vi "Test Configure.vi"(0 "Template Rx Test in":refnum<class "niDTS WLAN Rx Test.lvclass">, 11 "error in (no error)":errorcluster) -> (4 "Template Rx Test out":refnum<class "niDTS WLAN Rx Test.lvclass">, 15 "error out":errorcluster)   [LabVIEW 2015, in "niDTS WLAN.lvlib" / "niDTS WLAN Rx Test.lvclass"]
uses:
  niDTS WLAN Rx Test.lvclass
  niDTS WLAN Rx Test.lvclass/niDTS WLAN Rx Test.ctl
  RiviInstDriver/InstDriver/Objects/InstDriver.lvclass/InstDriver.ctl
  RiviInstDriver/InstDriver/Objects/Read VISA resource.vi
  TestStand/Station/Objects/SystemTechnologyCatalog/niDTS SystemTechnologyCatalog.lvclass
  TestStand/Station/Objects/SystemDut/niDTS SystemDut.lvclass
  Framework/Dut/Objects/BASE_class/niDTS Dut.lvclass
  Dut/Objects/BASE_class/niDTS WLAN Dut.lvclass
  Instrument/INSTR RX/niDTS WLAN INSTR RX.lvclass
  niDTS WLAN.lvlib
  Framework/niDTS Framework.lvlib
  RiviInstDriver/niRfsgWlan/Objects/niRfsgWlan.lvclass
  TestStand/niDTS TestStand.lvlib
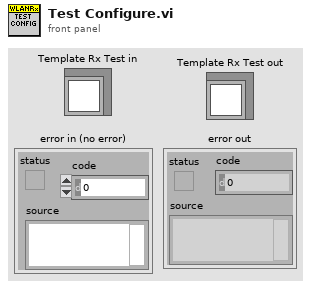
[diagram p1: front panel]
types:
  T1 = typedef "niDTS Framework.lvlib/niDTS Dut INC Handle.ctl" = refnum<data-value>
  T2 = typedef "niDTS WLAN.lvlib/niDTS WLAN Rx Test INC Parameters.ctl" = cluster{"Standard":T3, "DSSS Data Rate (Mbps)":T4, "OFDM Data Rate (Mbps)":T5, "MCS Index":i32, "N Spatial Streams":i32, "Chains":bool[], "Bandwidth (Hz)":T6, "Channel":i32, "Power (dBm)":dbl, "Guard Interval":T7, "FEC Coding":T8, "16 symbols":bool, "Payload Length (bytes)":i32, "Idle Interval (s)":dbl, "External Attenuation (dB)":dbl[], "RX Measurement Parameters":T9}
  T3 = typedef "niDTS WLAN.lvlib/niDTS WLAN INC Standard.ctl" = enum16{"802.11 b DSSS", "802.11 a/g OFDM", "802.11 n HT", "802.11 ac VHT"}
  T4 = typedef "niDTS WLAN.lvlib/niDTS WLAN INC DSSS Data Rate.ctl" = enum16{"1", "2", "5.5", "11"}
  T5 = typedef "niDTS WLAN.lvlib/niDTS WLAN INC OFDM Data Rate.ctl" = enum16{"6", "9", "12", "18", "24", "36", "48", "54"}
  T6 = typedef "niDTS WLAN.lvlib/niDTS WLAN INC CH BW.ctl" = enum16{"20 MHz", "40 MHz", "80 MHz", "160 MHz"}
  T7 = typedef "niDTS WLAN.lvlib/niDTS WLAN INC GI.ctl" = enum16{"LONG", "SHORT"}
  T8 = typedef "niDTS WLAN.lvlib/niDTS WLAN INC FEC Coding.ctl" = enum16{"BCC", "LDPC"}
  T9 = typedef "niDTS WLAN.lvlib/niDTS WLAN INC RX Measurement Parameters.ctl" = cluster{"Number of Packets":i32, "MacAddress":string}
  T10 = typedef "InstDriver.lvclass/niInstDriver INC Handle.ctl" = refnum<data-value>
  T11 = typedef "niDTS WLAN.lvlib/niDTS WLAN DUT INC Parameters.ctl" = cluster{"WLAN Type":T12, "Bandwidth (Hz)":T6, "Channel":i32, "Guard Interval":T7, "FEC Coding":T8, "Power (dBm)":dbl, "Payload Length (bytes)":i32, "16 Symbols":bool, "Chains":bool[]}
  T12 = typedef "niDTS WLAN.lvlib/niDTS WLAN INC Type.ctl" = enum16{"b - 1 Mbps", "b - 2 Mbps", "b - 5.5 Mbps", "b - 11 Mbps", "ag - 6 Mbps", "ag - 9 Mbps", "ag - 12 Mbps", "ag - 18 Mbps", "ag - 24 Mbps", "ag - 36 Mbps", "ag - 48 Mbps", "ag - 54 Mbps", "n - MCS0", "n - MCS1", "n - MCS2", "n - MCS3", "n - MCS4", "n - MCS5", "n - MCS6", "n - MCS7", "n - MCS8", "n - MCS9", "n - MCS10", "n - MCS11", "n - MCS12", "n - MCS13", "n - MCS14", "n - MCS15", "n - MCS16", "n - MCS17", "n - MCS18", "n - MCS19", "n - MCS20", "n - MCS21", "n - MCS22", "n - MCS23", "n - MCS24", "n - MCS25", "n - MCS26", "n - MCS27", "n - MCS28", "n - MCS29", "n - MCS30", "n - MCS31", "ac - MCS0 -1", "ac - MCS1 -1", "ac - MCS2 -1", "ac - MCS3 -1", "ac - MCS4 -1", "ac - MCS5 -1", "ac - MCS6 -1", "ac - MCS7 -1", "ac - MCS8 -1", "ac - MCS9 -1", "ac - MCS0 -2", "ac - MCS1 -2", "ac - MCS2 -2", "ac - MCS3 -2", "ac - MCS4 -2", "ac - MCS5 -2", "ac - MCS6 -2", "ac - MCS7 -2", "ac - MCS8 -2", "ac - MCS9 -2", "ac - MCS0 -3", "ac - MCS1 -3", "ac - MCS2 -3", "ac - MCS3 -3", "ac - MCS4 -3", "ac - MCS5 -3", "ac - MCS6 -3", "ac - MCS7 -3", "ac - MCS8 -3", "ac - MCS9 -3", "ac - MCS0 -4", "ac - MCS1 -4", "ac - MCS2 -4", "ac - MCS3 -4", "ac - MCS4 -4", "ac - MCS5 -4", "ac - MCS6 -4", "ac - MCS7 -4", "ac - MCS8 -4", "ac - MCS9 -4"}
  T13 = typedef "niDTS WLAN.lvlib/niDTS WLAN Dut INC Handle.ctl" = refnum<data-value>
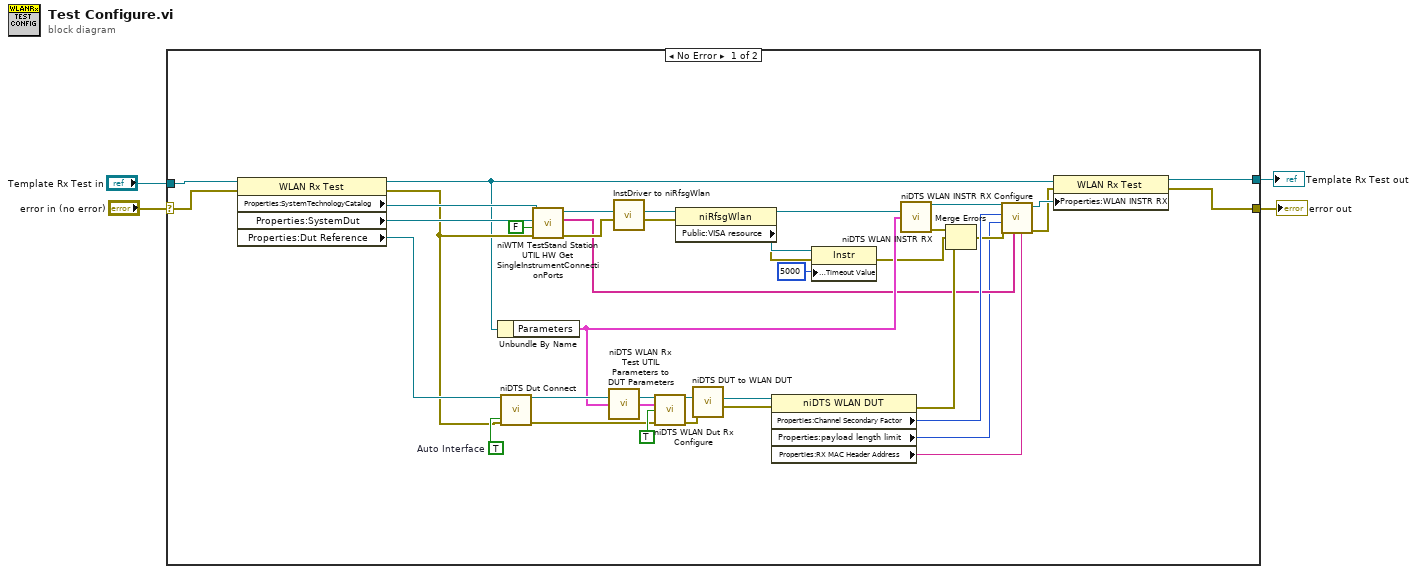
[diagram p0: block diagram]
diagram:
  n1 = case shown="No Error" "error in (no error)" {
    selector: "error in (no error)" -> [w43 w45]
    tunnel: [w40 w45] -> w2
    tunnel: [w41 w44] -> w3
    tunnel: "Template Rx Test in" -> [w42 w44]
    frame No Error {
      w38 = TRUE  # Auto Interface
      n2 = property class="WLAN Rx Test"(reference=w42, error in=w43) -> (reference out=w6:refnum<class "niDTS WLAN Rx Test.lvclass">, error out=w7:errorcluster, "Properties:SystemTechnologyCatalog"=w14:refnum<class "niDTS SystemTechnologyCatalog.lvclass">, "Properties:SystemDut"=w13:refnum<class "niDTS SystemDut.lvclass">, "Properties:Dut Reference"=w8:T1)
      n3 = Unbundle By Name(w6) -> ("Parameters"=w26:T2)
      n4 = call "niDTS Dut Connect.vi"("Dut Handle"=w8, "Auto Interface"=w38, "error in (no error)"=w7) -> ("Dut Handle out"=w37:T1, "error out"=w36:errorcluster)  [unwired: 11 in]
      n5 = call "niWTM TestStand Station UTIL HW Get SingleInstrumentConnectionPorts.vi"("error in (no error)"=w7, "TX Instrument"=FALSE, "SystemDut"=w13, "SystemTechnologyCatalog"=w14) -> ("error out"=w11:errorcluster, "Ports"=w10:string[], "InstDriver Handle"=w12:T10)  [unwired: 5 in]
      n6 = call "niDTS WLAN Rx Test UTIL Parameters to DUT Parameters.vi"("Parameters"=w26) -> ("TV Parameters(DataType)"=w28:T11)  [unwired: 14 in]
      n7 = call "InstDriver to niRfsgWlan.vi"("error in (no error)"=w11, "InstDriver Handle in"=w12) -> ("error out"=w34:errorcluster, "InstDriver Handle out"=w35:refnum<data-value>)  [unwired: 8 in]
      n8 = call "niDTS WLAN Dut Rx Configure.vi"("Dut Handle in"=w37, "niDTS WLAN DUT Parameters"=w28, "Apply Additional Defaults"=TRUE, "error in (no error)"=w36) -> ("Dut Handle"=w25:T1, "error out"=w24:errorcluster)  [unwired: 10 in]
      n9 = property class="niRfsgWlan"(reference=w35, error in=w34) -> (reference out=w30:refnum<data-value>, error out=w31:errorcluster, "Public:VISA resource"=w32:refnum<visa-resource-name>)
      n10 = call "niDTS DUT to WLAN DUT.vi"("error in"=w24, "Dut Handle"=w25) -> ("error out"=w23:errorcluster, "WLAN Dut Handle"=w27:T13)  [unwired: 8 in]
      n11 = property class="niDTS WLAN DUT"(reference=w27, error in=w23) -> (error out=w19:errorcluster, "Properties:Channel Secondary Factor"=w22:i8, "Properties:payload length limit"=w5:i32, "Properties:RX MAC Header Address"=w9:string)  [unwired: 1 out]
      n12 = property class="Instr"(reference=w32, error in=w31, "General Settings:Timeout Value"=u32 5000) -> (error out=w20:errorcluster)  [unwired: 1 out]
      n13 = call "niDTS WLAN INSTR RX.vi"("niRfsgWlan Handle"=w30, "WLAN Rx Input Parameters"=w26) -> ("niDTS WLAN INSTR RX"=w29:refnum<class "niDTS WLAN INSTR RX.lvclass">, "error out"=w21:errorcluster)  [unwired: 12 in]
      n14 = Merge Errors(w21, w20, w19) -> (w18:errorcluster)
      n15 = call-dynamic "niDTS WLAN INSTR RX Configure.vi"("MAC Address"=w9, "Port Names"=w10, "error in (no error)"=w18, "Payload length limit"=w5, "Channel Secondary Factor"=w22, "niDTS WLAN INSTR RX in"=w29) -> ("error out"=w16:errorcluster, "niDTS WLAN INSTR RX out"=w17:refnum<class "niDTS WLAN INSTR RX.lvclass">)  [unwired: 4 in]
      n16 = property class="WLAN Rx Test"(reference=w6, error in=w16, "Properties:WLAN INSTR RX"=w17) -> (reference out=w41:refnum<class "niDTS WLAN Rx Test.lvclass">, error out=w40:errorcluster)
    }
    frame Error {
    }
  }
  "error out" <- w2
  "Template Rx Test out" <- w3
